vi "Find Source Change.vi"(10 "New Value":cluster{"Channel":string, "Source":string}[](array[cluster]), 11 "Previous Value":cluster{"Channel":string, "Source":string}[](array[cluster])) -> (2 "Found?":bool, 3 "Item Index":i32)   [LabVIEW 2020, in "Routing and Faulting System Explorer.lvlib"]
uses:
  Routing and Faulting System Explorer.lvlib
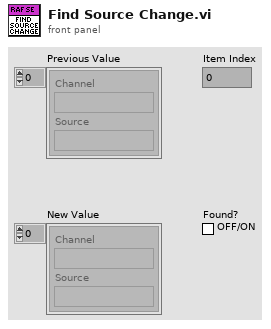
[diagram p1: front panel]
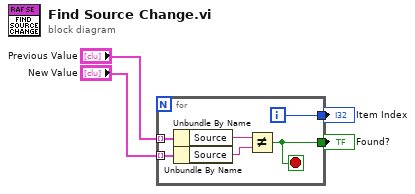
[diagram p0: block diagram]
diagram:
  n1 = for {
    tunnel: "Previous Value" -> [w10] mode=indexing
    tunnel: "New Value" -> [w9] mode=indexing
    tunnel: [w6] -> w2
    tunnel: [w5] -> w3
    i -> [w5]
    stop <- w6 stop-if-true
    n2 = Unbundle By Name(w10) -> ("Source"=w8:string)
    n3 = Unbundle By Name(w9) -> ("Source"=w7:string)
    n4 = Not Equal?(x=w8, y=w7) -> (x != y?=w6:bool)
  }
  "Item Index" <- w3
  "Found?" <- w2
